vi "标样核查数据组合(子VI).vi"(9 "小时数据发送次数":i32, 10 "数据输入":string[][](array[string]), 11 "污染物编码":string) -> (3 "输出组合":string)   [LabVIEW 2016, in "数据传输系统-04.lvlib"]
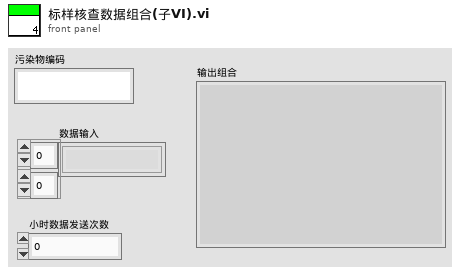
[diagram p1: front panel]
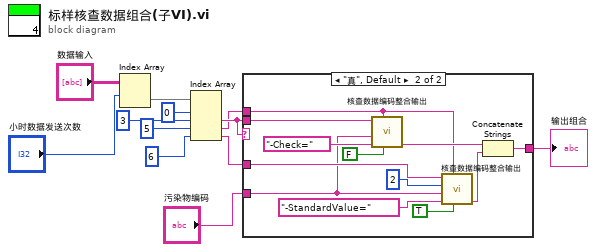
[diagram p0: block diagram]
diagram:
  n1 = Index Array(array="数据输入", index (row)="小时数据发送次数") -> (element=w10:string[])  [unwired: 1 in]
  n2 = Index Array(array=w10, index #1=0 ("索引"), index #2=3 ("索引"), index #3=5 ("索引"), index #4=6 ("索引")) -> (element #2=w7:string, element #3=w1:string, element #4=w4:string)  [unwired: 1 out]
  n3 = case shown="\"真\", Default" w7 {
    tunnel: w7 -> [w13 w25]
    tunnel: [w13 w22] -> w8
    tunnel: w4 -> [_ w19]
    tunnel: "污染物编码" -> [_ w15]
    tunnel: w1 -> [_ w14]
    frame "" {
    }
    frame "真", Default {
      n4 = call "核查数据编码整合输出.vi"("字段结束"=FALSE, "数据标识"=w14, "数据类型"="-Check=", "污染物编码"=w15, "数据值"=w25) -> ("编码输出"=w23:string)  [unwired: 6 in]
      n5 = call "核查数据编码整合输出.vi"("字段结束"=TRUE, "数据标识"=w14, "数据类型"="-StandardValue=", "污染物编码"=w15, "数据精度"=2, "数据值"=w19) -> ("编码输出"=w20:string)  [unwired: 5 in]
      n6 = Concatenate Strings(w23, w20) -> (w22:string)
    }
  }
  "输出组合" <- w8
